vi "Export the Data.vi"(8 "error in (no error)":errorcluster, 10 "File Format":string, 11 "Import Export in":refnum<class "Export.lvclass">) -> (0 "error out":errorcluster, 3 "Import Export out":refnum<class "Export.lvclass">)   [LabVIEW 2023, in "Data Analysis.lvlib" / "Export.lvlib" / "Export.lvclass"]
uses:
  Export.lvclass
  Export.lvclass/Export.ctl
  <vilib>/Utility/file.llb/Write Delimited Spreadsheet (string).vi
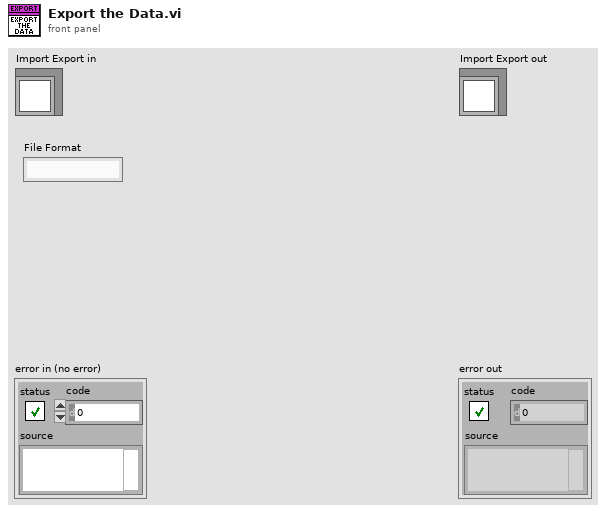
[diagram p1: front panel]
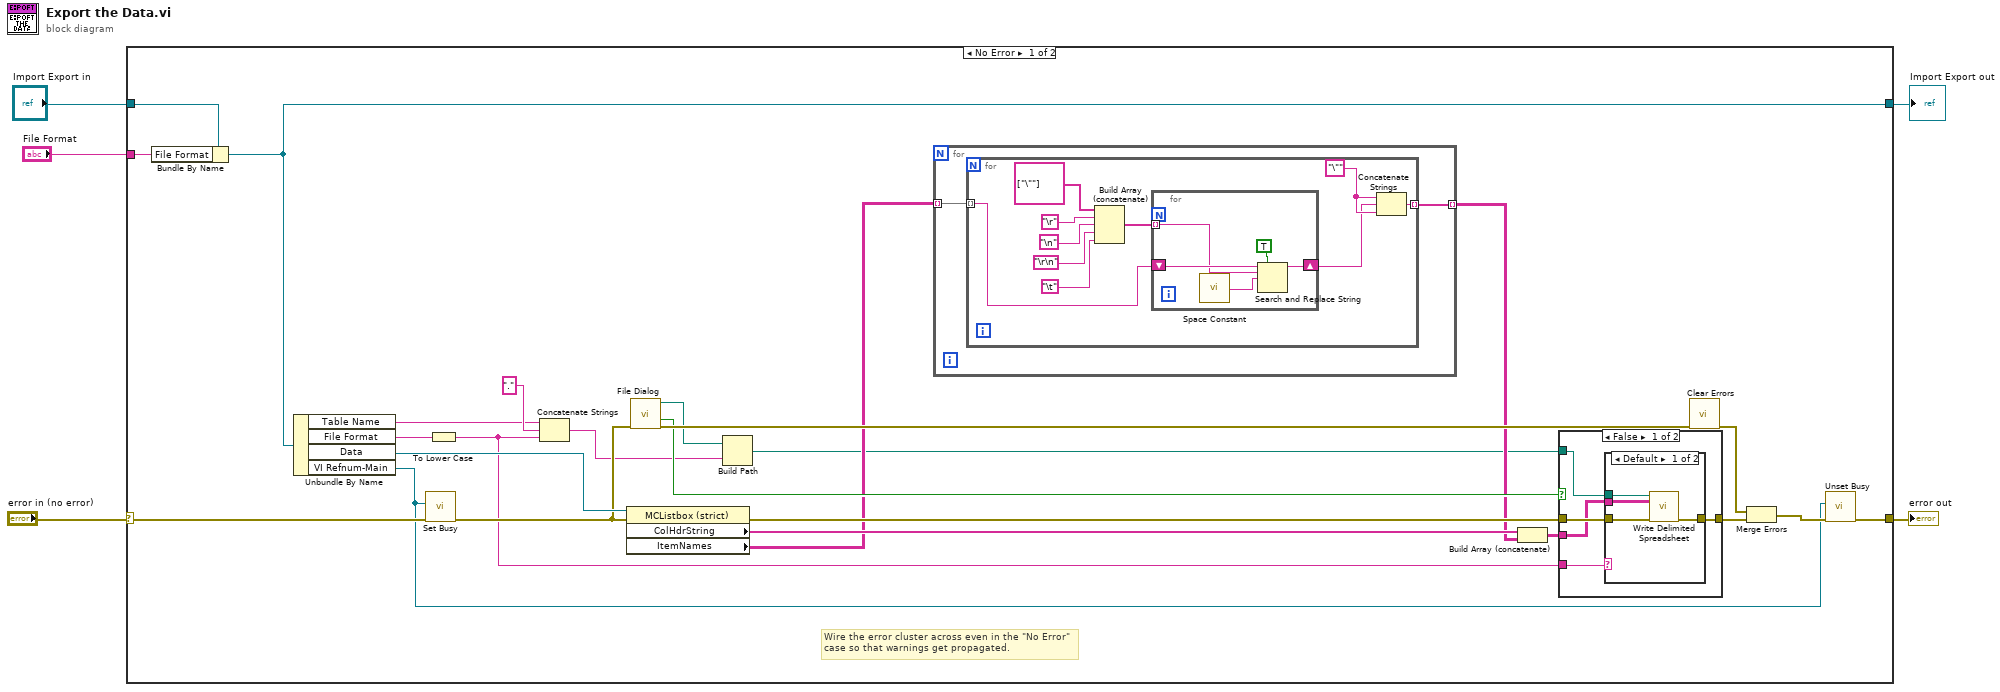
[diagram p0: block diagram]
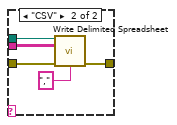
[diagram p2: hidden frame]
diagram:
  n1 = case shown="No Error" "error in (no error)" {
    selector: "error in (no error)" -> [w15 w64]
    tunnel: [w11 w64] -> w4
    tunnel: [w13 w63] -> w2
    tunnel: "Import Export in" -> [w18 w63]
    tunnel: "File Format" -> [w17 _]
    frame No Error {
      # "Wire the error cluster across even in the \"No Error\"\ncase so that warnings get propagated."
      n2 = Bundle By Name(cluster=w18, "File Format"=w17) -> (w13:refnum<class "Export.lvclass">)
      n3 = Unbundle By Name(w13) -> ("Table Name"=w8:string, "File Format"=w16:string, "Data"=w20:refnum<vi>, "VI Refnum-Main"=w10:refnum<vi>)
      n4 = call <vilib>:"Set Busy.vi"("error in (no error)"=w15, "VI reference (current VI)"=w10) -> ("error out"=w14:errorcluster)  [unwired: 8 in, 1 out]
      n5 = To Lower Case(string=w16) -> (all lower case string=w9:string)
      n6 = Concatenate Strings(w8, "." ("pattern (all files)"), w9) -> (w6:string)
      n7 = property class="MCListbox (strict)"(reference=w20, error in=w14) -> (error out=w30:errorcluster, "ColHdrString"=w25:string[], "ItemNames"=w24:string[][])  [unwired: 1 out]
      n8 = call "File Dialog"("error in"=w14) -> ("selected path"=w26:path, "cancelled"=w28:bool, "error out"=w29:errorcluster)  [unwired: 11 in, 1 out]
      n9 = Build Path(base path=w26, name or relative path=w6) -> (appended path=w7:path)
      n10 = for {
        tunnel: w24 -> [w32] mode=indexing
        tunnel: [w31] -> w23 mode=indexing
        n11 = for {
          tunnel: w32 -> [w34] mode=indexing
          tunnel: [w41] -> w31 mode=indexing
          w42 = "\""
          n12 = Build Array (concatenate)(string[] ["\""], "\r", "\n", "\r\n", "\t") -> (w40:string[])
          n13 = for {
            tunnel: w40 -> [w44] mode=indexing
            shift-right: [w45] -> w33
            shift-left: w34 -> [w46]
            n14 = call <vilib>:"Space Constant.vi"() -> ("String"=w43:string)
            n15 = Search and Replace String(replace all?=TRUE ("replace all? (F)"), input string=w46, search string=w44, replace string=w43) -> (result string=w45:string)  [unwired: 4 in, 3 out]
          }
          n16 = Concatenate Strings(w42, w33, w42) -> (w41:string)
        }
      }
      n17 = Build Array (concatenate)(w25, w23) -> (w27:string[][])
      n18 = case shown="False" w28 {
        tunnel: w30 -> [w52 w62]
        tunnel: [w51 w62] -> w22
        tunnel: w27 -> [w50 _]
        tunnel: w7 -> [w49 _]
        tunnel: w9 -> [w48 _]
        frame False {
          n19 = case shown="Default" w48 {
            tunnel: w52 -> [w56 w61]
            tunnel: [w55 w60] -> w51
            tunnel: w50 -> [w54 w59]
            tunnel: w49 -> [w53 w58]
            frame Default {
              n20 = call-poly <vilib>:"Write Delimited Spreadsheet.vi"("file path (dialog if empty)"=w53, "2D data"=w54, "error in (no error)"=w56) -> ("error out"=w55:errorcluster)  [unwired: 11 in, 1 out]
            }
            frame "CSV" {
              n21 = call-poly <vilib>:"Write Delimited Spreadsheet.vi"("file path (dialog if empty)"=w58, "2D data"=w59, "error in (no error)"=w61, "delimiter (\\t)"="," ("delimiter (\\t)")) -> ("error out"=w60:errorcluster)  [unwired: 10 in, 1 out]
            }
          }
        }
        frame True {
        }
      }
      n22 = call <vilib>:"Clear Errors.vi"("error in (no error)"=w29) -> ("error out"=w21:errorcluster)  [unwired: 5 in, 1 out]
      n23 = Merge Errors(w21, w22) -> (w12:errorcluster)
      n24 = call <vilib>:"Unset Busy.vi"("error in (no error)"=w12, "VI reference (current VI)"=w10) -> ("error out"=w11:errorcluster)  [unwired: 9 in]
    }
    frame Error {
    }
  }
  "error out" <- w4
  "Import Export out" <- w2
